vi "cout+.vi"(2 "I":dbl[][](array[numeric]), 3 "<B>":dbl, 4 "B":dbl[](array[numeric]), 5 "采样点数":i32) -> (0 "N+":dbl, 1 "I'":dbl[][](array[numeric]))   [LabVIEW 2018]
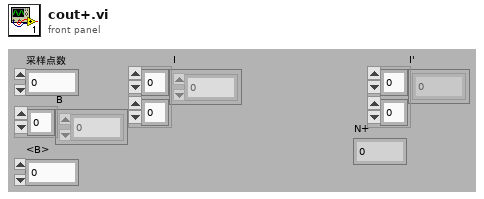
[diagram p1: front panel]
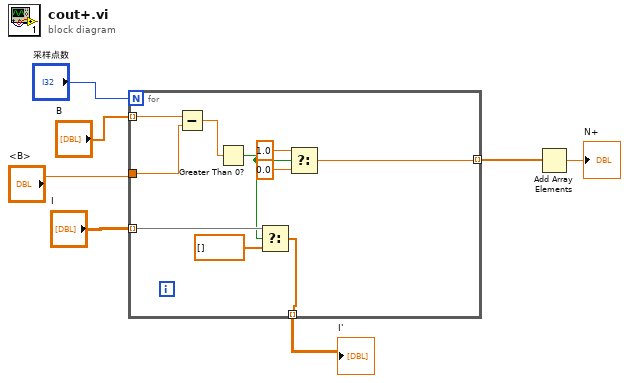
[diagram p0: block diagram]
diagram:
  n1 = for {
    N: "采样点数" -> [_]
    tunnel: "B" -> [w17] mode=indexing
    tunnel: "<B>" -> [w16]
    tunnel: "I" -> [w15] mode=indexing
    tunnel: [w13] -> w3 mode=indexing
    tunnel: [w8] -> w2 mode=indexing
    n2 = Subtract(x=w17, y=w16) -> (x-y=w12:dbl)
    n3 = Greater Than 0?(x=w12) -> (x > 0?=w11:bool)
    n4 = Select(t=w15, s=w11, f=dbl[] []) -> (s? t:f=w13:dbl[])
    n5 = Select(t=1.0, s=w11, f=0.0) -> (s? t:f=w8:dbl)
  }
  "I'" <- w3
  n6 = Add Array Elements(numeric array=w2) -> (sum=→"N+":dbl)
